vi "Clear Tree.vi"(8 "Error In":errorcluster, 11 "State In":T1) -> (0 "Error Out":errorcluster, 3 "State Out":T1)   [LabVIEW 2017, in "Eulogy.lvlib" / "Bookmark Manager.lvlib"]
uses:
  Bookmark Manager.lvlib
  State.ctl
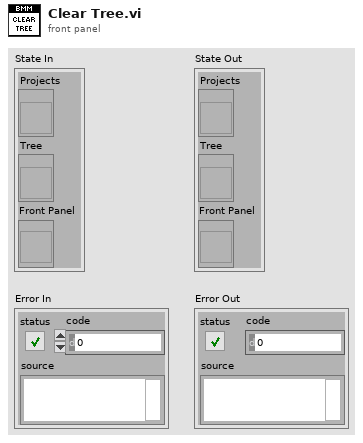
[diagram p1: front panel]
types:
  T1 = typedef "Eulogy.lvlib/Bookmark Manager.lvlib/State.ctl" = cluster{"Projects":refnum<vi>, "Tree":refnum<vi>, "Front Panel":refnum<vi>}
  T2 = enum8{"Enabled", "Disabled", "Disabled and Grayed Out"}
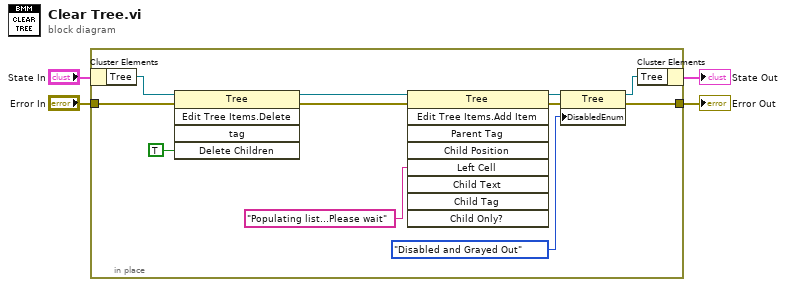
[diagram p0: block diagram]
diagram:
  n1 = in-place {
    in-place-border: "Error In" -> [w6]
    in-place-border: [w5] -> w4
    n2 = in-place-cluster #1("State In") -> ("Tree"=w8:refnum<vi>)
    n3 = invoke class="Tree" method="Edit Tree Items.Delete"(reference=w8, error in=w6, "Delete Children"=TRUE ("Delete Children?")) -> (reference out=w14:refnum<vi>, error out=w13:errorcluster)  [unwired: 2 in, 3 out]
    n4 = invoke class="Tree" method="Edit Tree Items.Add Item"(reference=w14, error in=w13, "Left Cell"="Populating list...Please wait" ("Left Cell String")) -> (reference out=w11:refnum<vi>, error out=w10:errorcluster)  [unwired: 6 in, 7 out]
    n5 = property class="Tree"(reference=w11, error in=w10, "DisabledEnum"=T2."Disabled and Grayed Out" ("Disabled")) -> (reference out=w7:refnum<vi>, error out=w5:errorcluster)
    n6 = in-place-cluster #1("Tree"=w7) -> (→"State Out":T1)
  }
  "Error Out" <- w4
